vi "Avante_shift.vi"() -> ()   [LabVIEW 2015]
uses:
  <vilib>/National Instruments/NI Dynamixel API/Dynamixel Pro Driver/Controls/Write Select Pro.ctl
  <vilib>/National Instruments/NI Dynamixel API/Dynamixel Pro Driver/Controls/Baudrate Selector.ctl
  G_ALL.vi
  <vilib>/National Instruments/NI Dynamixel API/Dynamixel Pro Driver/Write/Write Dynamixel Pro.vi
  <vilib>/National Instruments/NI Dynamixel API/Dynamixel Pro Driver/Helper VIs/Torque Disable.vi
  <vilib>/National Instruments/NI Dynamixel API/Dynamixel Pro Driver/Helper VIs/Torque Enable.vi
  <vilib>/National Instruments/NI Dynamixel API/Dynamixel Pro Driver/Dynamixel Pro Driver.lvlib
panel:
  out "robotis":refnum<visa-resource-name>
  in  "gain":i32=50
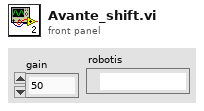
[diagram p1: front panel]
types:
  T1 = typedef "Dynamixel Pro Driver.lvlib/Write Select Pro.ctl" = enum16{"ID", "Baud Rate", "Return Delay Time", "Operating mode", "Homing offset", "Moving threshold", "Temperature limit", "Max Voltage Limit", "Min Voltage Limit", "acceleration Limit", "Torque Limit", "Velocity Limit", "Max Position Limit", "Min Position Limit", "External Port Mode 1", "External Port Mode 2", "External Port Mode 3", "External Port Mode 4", "Shutdown", "Torque Enable", "LED RED", "LED GREEN", "LED BLUE", "Velocity I Gain", "Velocity P Gain", "Position P Gain", "Goal Position", "Goal Velocity", "Goal Torque", "Goal Acceleration", "External Port Data 1", "External Port Data 2", "External Port Data 3", "External Port Data 4", "Status Return Level"}
  T2 = typedef "Dynamixel Pro Driver.lvlib/Baudrate Selector.ctl" = enum16{"2400", "57600", "115200", "1000000", "2000000", "3000000", "4000000", "4500000", "10500000"}
  T3 = cluster{"Steer_input":dbl, "Steer_output":dbl, "VS_des":dbl, "VS_can":dbl, "heading":dbl, "auto":bool, "run":bool, "x":dbl, "y":dbl}
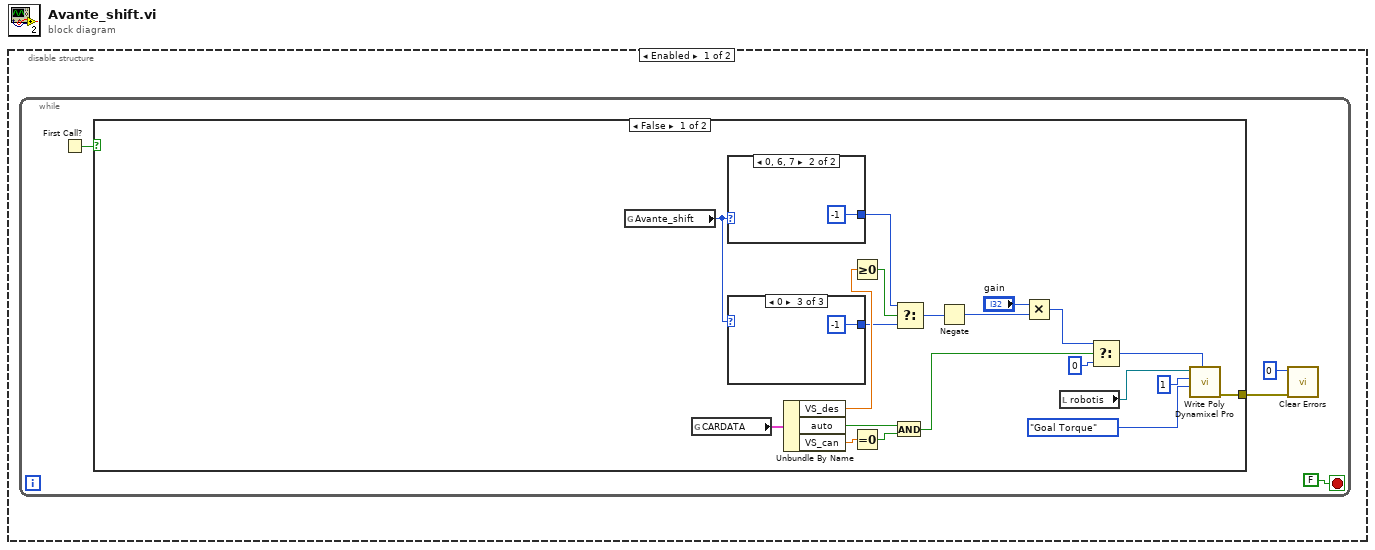
[diagram p0: block diagram]
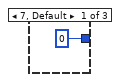
[diagram p2: hidden frame]
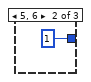
[diagram p3: hidden frame]
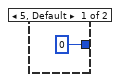
[diagram p4: hidden frame]
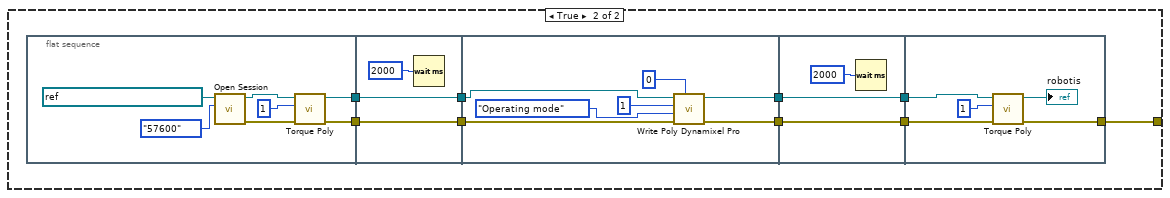
[diagram p5: hidden frame]
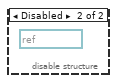
[diagram p6: hidden frame]
diagram:
  n1 = disable-structure shown="Enabled" {
    frame Enabled {
      n2 = while {
        stop <- FALSE ("status") stop-if-true
        n3 = First Call?() -> (First Call?: T/F=w4:bool)
        n4 = case shown="False" w4 {
          tunnel: [w24 w30] -> w3
          frame False {
            n5 = global read "G_ALL.vi" "Avante_shift"() -> (w12:u8)
            n6 = global read "G_ALL.vi" "CARDATA"() -> (w17:T3)
            n7 = case shown="0, 6, 7" w12 {
              tunnel: [0 -1] -> w10
              frame 5, Default {
              }
              frame 0, 6, 7 {
              }
            }
            n8 = case shown="0" w12 {
              tunnel: [0 1 -1] -> w9
              frame 7, Default {
              }
              frame 5, 6 {
              }
              frame 0 {
              }
            }
            n9 = Unbundle By Name(w17) -> ("VS_des"=w13:dbl, "auto"=w15:bool, "VS_can"=w16:dbl)
            n10 = Greater Or Equal To 0?(x=w13) -> (x >= 0?=w11:bool)
            n11 = Equal To 0?(x=w16) -> (x = 0?=w14:bool)
            n12 = And(x=w15, y=w14) -> (x .and. y?=w23:bool)
            n13 = Select(t=w10, s=w11, f=w9) -> (s? t:f=w8:i32)
            n14 = Negate(x=w8) -> (-x=w7:i32)
            n15 = Multiply(x="gain", y=w7) -> (x*y=w19:i32)
            n16 = local read "robotis"() -> (w5:refnum<visa-resource-name>)
            n17 = Select(t=w19, s=w23, f=0) -> (s? t:f=w20:i32)
            n18 = call-poly <vilib>:"Write Poly Dynamixel Pro.vi"("Value"=w20, "Operation"=Write_Select_Pro."Goal Torque", "ID"=u8 1, "VISA Refnum in"=w5) -> ("error out"=w24:errorcluster)  [unwired: 6 in, 1 out]
          }
          frame True {
            n19 = flat-sequence {
              tunnel: [w41] -> w38
              tunnel: [w40] -> w37
              tunnel: [w48] -> w36
              tunnel: w38 -> [w48]
              tunnel: [w47] -> w35
              tunnel: w37 -> [w47]
              tunnel: [w52] -> w34
              tunnel: w36 -> [w54]
              tunnel: w35 -> [w53]
              tunnel: [w51] -> w33
              tunnel: w34 -> [w58]
              tunnel: [w58] -> w32
              tunnel: [w57] -> w31
              tunnel: w33 -> [w57]
              tunnel: [w61] -> w30
              tunnel: w32 -> [w63]
              tunnel: w31 -> [w62]
              frame #0 {
                n20 = call <vilib>:"Open Session.vi"("Baud Rate"=Baudrate_Selector."57600", "VISA resource name"=refnum<visa-resource-name> "COM5") -> ("error out"=w44:errorcluster, "VISA Refnum out"=w45:refnum<visa-resource-name>)  [unwired: 8 in]
                n21 = call-poly <vilib>:"Torque Poly.vi"("error in (no error)"=w44, "ID"=u8 1, "VISA Refnum in"=w45) -> ("error out"=w40:errorcluster, "VISA Refnum out"=w41:refnum<visa-resource-name>)  [unwired: 7 in]
              }
              frame #1 {
                n22 = Wait (ms)(milliseconds to wait=u32 2000) -> ()  [unwired: 1 out]
              }
              frame #2 {
                n23 = call-poly <vilib>:"Write Poly Dynamixel Pro.vi"("Value"=0, "error in (no error)"=w53, "Operation"=Write_Select_Pro."Operating mode", "ID"=u8 1, "VISA Refnum in"=w54) -> ("error out"=w51:errorcluster, "VISA Refnum out"=w52:refnum<visa-resource-name>)  [unwired: 5 in]
              }
              frame #3 {
                n24 = Wait (ms)(milliseconds to wait=u32 2000) -> ()  [unwired: 1 out]
              }
              frame #4 {
                n25 = call-poly <vilib>:"Torque Poly.vi"("error in (no error)"=w62, "ID"=u8 1, "VISA Refnum in"=w63) -> ("error out"=w61:errorcluster, "VISA Refnum out"=→"robotis":refnum<visa-resource-name>)  [unwired: 7 in]
              }
            }
          }
        }
        n26 = call <vilib>:"Clear Errors.vi"("error in (no error)"=w3, "specific error code to clear (0: all)"=0) -> ()  [unwired: 4 in, 2 out]
      }
    }
    frame Disabled {
      w64 = refnum<visa-resource-name> "COM5" ("VISA resource name")
    }
  }
